vi "RecordTrig_DerotatorControl.vi"() -> ()   [LabVIEW 2021]
uses:
  <vilib>/DAQmx/write.llb/DAQmx Write (Digital Bool 1Line 1Point).vi
  <vilib>/DAQmx/create/channels.llb/DAQmx Create Channel (DO-Digital Output).vi
  <vilib>/DAQmx/miscellaneous.llb/DAQmx Fill In Error Info.vi
panel:
  in  "pulse wait":u32=50
  in  "Move Derotator":bool
  in  "Direction":bool
  in  "stop":bool
  in  "Record!":bool
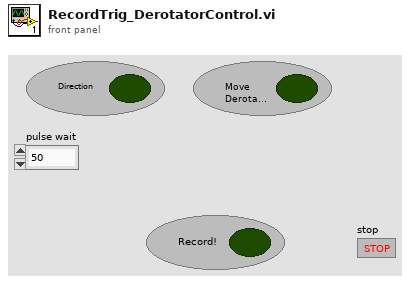
[diagram p1: front panel]
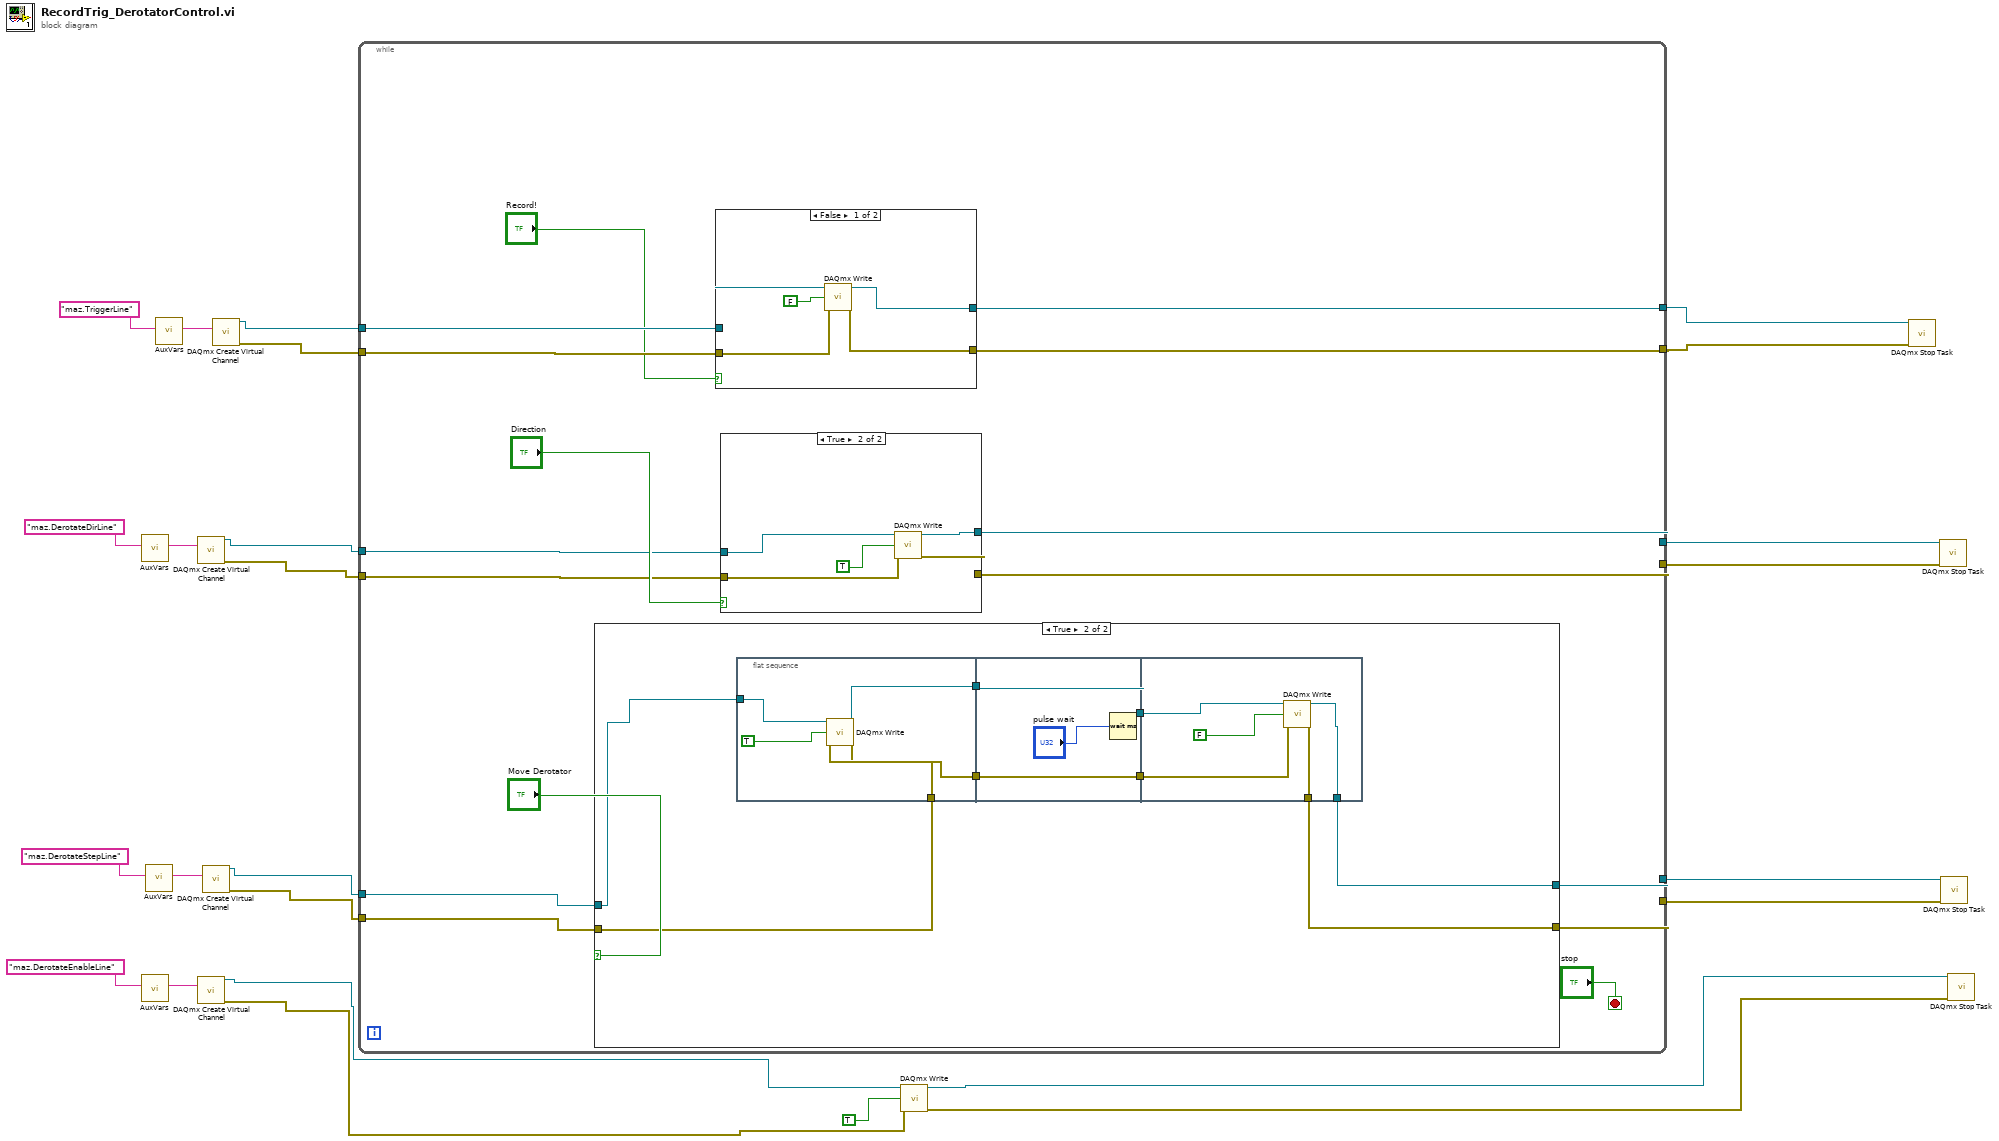
[diagram p0: block diagram]
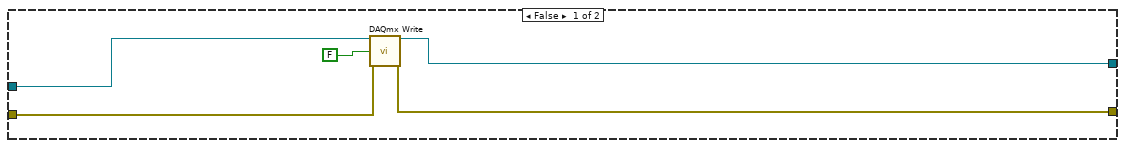
[diagram p2: hidden frame]
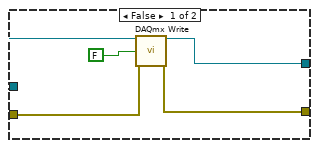
[diagram p3: hidden frame]
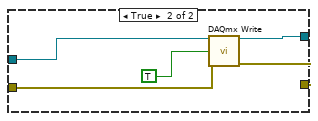
[diagram p4: hidden frame]
diagram:
  n1 = call "AuxVars.vi"("key"="maz.DerotateDirLine") -> ("value"=w19:string)  [unwired: 9 in, 1 out]
  n2 = call "AuxVars.vi"("key"="maz.DerotateEnableLine") -> ("value"=w15:string)  [unwired: 9 in, 1 out]
  n3 = call "AuxVars.vi"("key"="maz.DerotateStepLine") -> ("value"=w17:string)  [unwired: 9 in, 1 out]
  n4 = call "AuxVars.vi"("key"="maz.TriggerLine") -> ("value"=w25:string)  [unwired: 9 in, 1 out]
  n5 = call-poly <vilib>:"DAQmx Create Virtual Channel.vi"("lines"=w19) -> ("task out"=w9:refnum<k21>, "error out"=w8:errorcluster)  [unwired: 13 in]
  n6 = call-poly <vilib>:"DAQmx Create Virtual Channel.vi"("lines"=w15) -> ("task out"=w4:refnum<k21>, "error out"=w1:errorcluster)  [unwired: 13 in]
  n7 = call-poly <vilib>:"DAQmx Create Virtual Channel.vi"("lines"=w17) -> ("task out"=w13:refnum<k21>, "error out"=w12:errorcluster)  [unwired: 13 in]
  n8 = call-poly <vilib>:"DAQmx Create Virtual Channel.vi"("lines"=w25) -> ("task out"=w23:refnum<k21>, "error out"=w22:errorcluster)  [unwired: 13 in]
  n9 = while {
    tunnel: w23 -> [w41]
    tunnel: w22 -> [w40]
    tunnel: [w39] -> w21
    tunnel: [w38] -> w20
    tunnel: w13 -> [w33]
    tunnel: w12 -> [w32]
    tunnel: [w31] -> w11
    tunnel: [w30] -> w10
    tunnel: w9 -> [w29]
    tunnel: w8 -> [w28]
    tunnel: [w27] -> w7
    tunnel: [w26] -> w6
    stop <- "stop" stop-if-true
    n10 = case shown="True" "Move Derotator" {
      tunnel: w33 -> [w45 w54]
      tunnel: w32 -> [w44 w53]
      tunnel: [w43 w47] -> w30
      tunnel: [w42 w48] -> w31
      frame False {
        n11 = call-poly <vilib>:"DAQmx Write.vi"("task/channels in"=w45, "data"=FALSE, "error in"=w44) -> ("task out"=w43:refnum<k21>, "error out"=w42:errorcluster)  [unwired: 10 in, 1 out]
      }
      frame True {
        n12 = flat-sequence {
          tunnel: w54 -> [w59]
          tunnel: w53 -> [w58]
          tunnel: [w57] -> w52
          tunnel: [w55] -> w50
          tunnel: w52 -> [w62]
          tunnel: [w62] -> w51
          tunnel: w50 -> [w60]
          tunnel: [w60] -> w49
          tunnel: w51 -> [w67]
          tunnel: w49 -> [w65]
          tunnel: [w64] -> w48
          tunnel: [w63] -> w47
          frame #0 {
            n13 = call-poly <vilib>:"DAQmx Write.vi"("task/channels in"=w59, "data"=TRUE, "error in"=w58) -> ("task out"=w57:refnum<k21>, "error out"=w55:errorcluster)  [unwired: 10 in, 1 out]
          }
          frame #1 {
            n14 = Wait (ms)(milliseconds to wait="pulse wait") -> ()  [unwired: 1 out]
          }
          frame #2 {
            n15 = call-poly <vilib>:"DAQmx Write.vi"("task/channels in"=w67, "data"=FALSE, "error in"=w65) -> ("task out"=w63:refnum<k21>, "error out"=w64:errorcluster)  [unwired: 10 in, 1 out]
          }
        }
      }
    }
    n16 = case shown="False" "Record!" {
      tunnel: w41 -> [w81 w87]
      tunnel: w40 -> [w80 w86]
      tunnel: [w79 w85] -> w39
      tunnel: [w78 w84] -> w38
      frame False {
        n17 = call-poly <vilib>:"DAQmx Write.vi"("task/channels in"=w81, "data"=FALSE, "error in"=w80) -> ("task out"=w79:refnum<k21>, "error out"=w78:errorcluster)  [unwired: 10 in, 1 out]
      }
      frame True {
        n18 = call-poly <vilib>:"DAQmx Write.vi"("task/channels in"=w87, "data"=TRUE, "error in"=w86) -> ("task out"=w85:refnum<k21>, "error out"=w84:errorcluster)  [unwired: 10 in, 1 out]
      }
    }
    n19 = case shown="True" "Direction" {
      tunnel: w29 -> [w71 w77]
      tunnel: w28 -> [w70 w76]
      tunnel: [w69 w75] -> w26
      tunnel: [w68 w74] -> w27
      frame False {
        n20 = call-poly <vilib>:"DAQmx Write.vi"("task/channels in"=w71, "data"=FALSE, "error in"=w70) -> ("task out"=w69:refnum<k21>, "error out"=w68:errorcluster)  [unwired: 10 in, 1 out]
      }
      frame True {
        n21 = call-poly <vilib>:"DAQmx Write.vi"("task/channels in"=w77, "data"=TRUE, "error in"=w76) -> ("task out"=w75:refnum<k21>, "error out"=w74:errorcluster)  [unwired: 10 in, 1 out]
      }
    }
  }
  n22 = call-poly <vilib>:"DAQmx Write.vi"("task/channels in"=w4, "data"=TRUE, "error in"=w1) -> ("task out"=w3:refnum<k21>, "error out"=w2:errorcluster)  [unwired: 10 in, 1 out]
  n23 = call <vilib>:"DAQmx Stop Task.vi"("task/channels in"=w21, "error in"=w20) -> ()  [unwired: 12 in, 2 out]
  n24 = call <vilib>:"DAQmx Stop Task.vi"("task/channels in"=w6, "error in"=w7) -> ()  [unwired: 12 in, 2 out]
  n25 = call <vilib>:"DAQmx Stop Task.vi"("task/channels in"=w10, "error in"=w11) -> ()  [unwired: 12 in, 2 out]
  n26 = call <vilib>:"DAQmx Stop Task.vi"("task/channels in"=w3, "error in"=w2) -> ()  [unwired: 12 in, 2 out]
